vi "GetNavigationInProgress.vi"(8 "error in (no error)":errorcluster, 11 "AbstractWorldMap in":refnum<class "NI_Robotics_AbstractWorldMap.lvclass">) -> (0 "error out":errorcluster, 2 "Navigation in Progress":bool, 3 "AbstractWorldMap out":refnum<class "NI_Robotics_AbstractWorldMap.lvclass">)   [LabVIEW 2017, in "NI_Robotics_AbstractWorldMap.lvclass"]
uses:
  <vilib>/robotics/Navigation/shared/WorldMap/AbstractWorldMap/NI_Robotics_AbstractWorldMap.lvclass
  <vilib>/robotics/Navigation/shared/WorldMap/AbstractWorldMap/NI_Robotics_AbstractWorldMap.lvclass/NI_Robotics_AbstractWorldMap.ctl
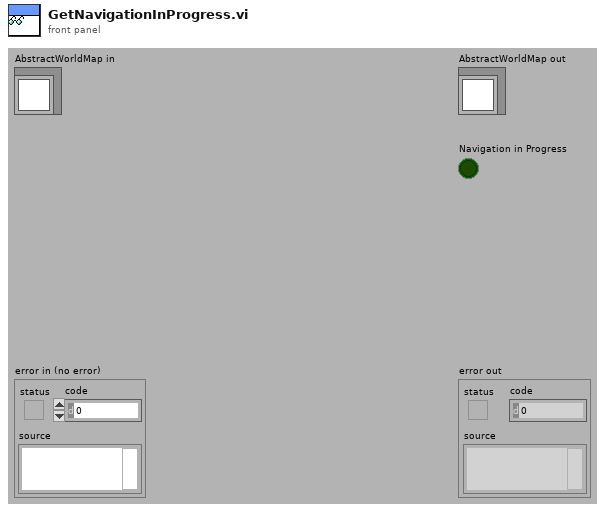
[diagram p1: front panel]
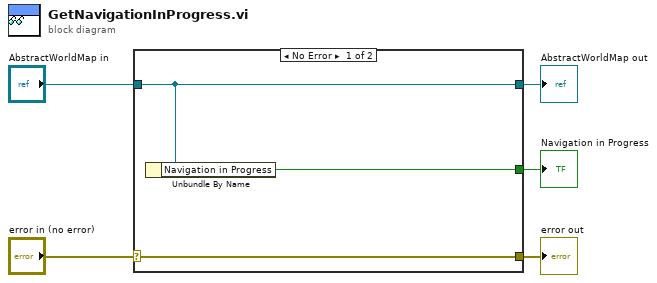
[diagram p0: block diagram]
diagram:
  n1 = case shown="No Error" "error in (no error)" {
    selector: "error in (no error)" -> [w8 w9]
    tunnel: [w8 w9] -> w4
    tunnel: [w7 w10] -> w2
    tunnel: "AbstractWorldMap in" -> [w7 w10]
    tunnel: [w6 _] -> w1
    frame No Error {
      n2 = Unbundle By Name(w7) -> ("Navigation in Progress"=w6:bool)
    }
    frame Error {
    }
  }
  "error out" <- w4
  "AbstractWorldMap out" <- w2
  "Navigation in Progress" <- w1
